vi "Copie de SaveTempData2.vi"(2 "temp data":dbl[][][](array[numeric]), 3 "Exp_params":T3={"filename"="201612011532", "ExpFilePath"=path "\\\\10.0.0.7\\takada2/DATA/HBT6/data/Test/201612011532.h5", "File Ref list"=[16777216, 33554432], "sweep_dim"=[4, 2], "sweep_list"=[], "readout_list"=["ADC0", "ADC1"], "Sweep instrument bools"=[[0, 0], [0, 0], [0, 0], [0, 0], [0, 0], [0, 0], [0, 0], [0, 0], [0, 0], [0, 0], [0, 0], [0, 0], [0, 0], [0, 0], [0, 0], [0, 0], [0, 0], [0, 0], [0, 0], [0, 0], [0, 0], [0, 0], [0, 0], [0, 0], [0, 0], [0, 0], [0, 0], [0, 0], [0, 0], [0, 0], [0, 0]], "Read out instrument bools"=[[1, 0]], "Experimental bool list"=[FALSE, TRUE], "Initial move"=[{"Name"="None", "kind"=100, "Value"=0.0}], "FPGA Ref"=refnum, "Inst_parameters"={"ConfigFilePath"=path "\\\\10.0.0.7\\takada2/DATA/HBT6/data/Configs/HBT6_ramp_1.h5", "Inst_list"=["ADC", "AWG", "Freq", "Power", "sus", "rus", "rls", "sls", "suq", "suu", "sur", "suc", "sul", "ruq", "ruu", "rur", "ruc", "rul", "rlq", "rlu", "rlr", "rlc", "rll", "slq", "slu", "slr", "slc", "sll", "tu", "t", "tl", "fast_sequence"], "fast_mode"=[1, 1], "Wait_times"=[1, 1, 1, 1], "Inst_array"=[{"Kind"=0, "Strings"=["ADC", "", "V", "ADC0;ADC1", "V;V", "1.0;1.0"], "uint64s"=[10, 2, 250000, 0, 100, 10106, 1000000, 1, 0, 1], "Doubles"=[1.0], "DAQmx take out list"=[]}, {"Kind"=7, "Strings"=["AWG", "10.0.0.4", "", "C:\\Documents and Settings\\Bauerle\\Mes documents\\Bautze\\FPGA-clean_works_1.13.6_batchtest\\Python\\AWG", "dummy", "SAWnstrig_v4.py"], "uint64s"=[2, 0, 0, 3, 0, 0, 0, 0, 0, 0, 0, 0, 0, 0], "Doubles"=[1200000000.0, 1.0, 0.0, 1.0, 0.0, 1.0, 0.0, 1.0, 0.0, 1.0, 0.0, 1.0, 0.0], "DAQmx take out list"=[]}, {"Kind"=6, "Strings"=["Freq", "0:19", "GHz"], "uint64s"=[1, 0, 0, 0, 2, 0, 0, 0], "Doubles"=[2.0, -30.0, 200.0, 100.0, 0.0, 6.000999927520752, 9.000000318337698e-06, 30.0, -145.0], "DAQmx take out list"=[]}, {"Kind"=6, "Strings"=["Power", "0:19", "GHz"], "uint64s"=[1, 0, 1, 0, 2, 0, 0, 0], "Doubles"=[2.0, -30.0, 200.0, 100.0, 0.0, 6.000999927520752, 9.000000318337698e-06, 30.0, -145.0], "DAQmx take out list"=[]}, {"Kind"=4, "Strings"=["sus", "10.0.0.2", "mV"], "uint64s"=[0, 1], "Doubles"=[1.0, -1.0, 1.0, -1.0, 1.0], "DAQmx take out list"=[]}, {"Kind"=4, "Strings"=["rus", "10.0.0.2", "mV"], "uint64s"=[0, 2], "Doubles"=[1.0, -1.0, 1.0, -1.0, 1.0], "DAQmx take out list"=[]}, {"Kind"=4, "Strings"=["rls", "10.0.0.2", "mV"], "uint64s"=[0, 3], "Doubles"=[1.0, -1.0, 1.0, -1.0, 1.0], "DAQmx take out list"=[]}, {"Kind"=4, "Strings"=["sls", "10.0.0.2", "mV"], "uint64s"=[0, 4], "Doubles"=[1.0, -1.0, 1.0, -1.0, 1.0], "DAQmx take out list"=[]}, {"Kind"=4, "Strings"=["suq", "10.0.0.2", "V"], "uint64s"=[0, 5], "Doubles"=[0.30000001192092896, -2.0, 1.0, -1.0, 1.0], "DAQmx take out list"=[]}, {"Kind"=4, "Strings"=["suu", "10.0.0.2", "V"], "uint64s"=[0, 6], "Doubles"=[0.30000001192092896, -2.0, 1.0, -1.0, 1.0], "DAQmx take out list"=[]}, {"Kind"=4, "Strings"=["sur", "10.0.0.2", "V"], "uint64s"=[0, 7], "Doubles"=[0.30000001192092896, -2.0, 1.0, -1.0, 1.0], "DAQmx take out list"=[]}, {"Kind"=4, "Strings"=["suc", "10.0.0.2", "V"], "uint64s"=[1, 0], "Doubles"=[0.30000001192092896, -2.0, 1.0, -1.0, 1.0], "DAQmx take out list"=[]}, {"Kind"=4, "Strings"=["sul", "10.0.0.2", "V"], "uint64s"=[1, 1], "Doubles"=[0.30000001192092896, -2.0, 1.0, -1.0, 1.0], "DAQmx take out list"=[]}, {"Kind"=4, "Strings"=["ruq", "10.0.0.2", "V"], "uint64s"=[1, 2], "Doubles"=[0.30000001192092896, -2.0, 1.0, -1.0, 1.0], "DAQmx take out list"=[]}, {"Kind"=4, "Strings"=["ruu", "10.0.0.2", "V"], "uint64s"=[1, 3], "Doubles"=[0.30000001192092896, -2.0, 1.0, -1.0, 1.0], "DAQmx take out list"=[]}, {"Kind"=4, "Strings"=["rur", "10.0.0.2", "V"], "uint64s"=[1, 5], "Doubles"=[0.30000001192092896, -2.0, 1.0, -1.0, 1.0], "DAQmx take out list"=[]}, {"Kind"=4, "Strings"=["ruc", "10.0.0.2", "V"], "uint64s"=[1, 6], "Doubles"=[0.30000001192092896, -2.0, 1.0, -1.0, 1.0], "DAQmx take out list"=[]}, {"Kind"=4, "Strings"=["rul", "10.0.0.2", "V"], "uint64s"=[1, 7], "Doubles"=[0.30000001192092896, -2.0, 1.0, -1.0, 1.0], "DAQmx take out list"=[]}, {"Kind"=4, "Strings"=["rlq", "10.0.0.2", "V"], "uint64s"=[2, 0], "Doubles"=[0.30000001192092896, -2.0, 1.0, -1.0, 1.0], "DAQmx take out list"=[]}, {"Kind"=4, "Strings"=["rlu", "10.0.0.2", "V"], "uint64s"=[2, 1], "Doubles"=[0.30000001192092896, -2.0, 1.0, -1.0, 1.0], "DAQmx take out list"=[]}, {"Kind"=4, "Strings"=["rlr", "10.0.0.2", "V"], "uint64s"=[2, 2], "Doubles"=[0.30000001192092896, -2.0, 1.0, -1.0, 1.0], "DAQmx take out list"=[]}, {"Kind"=4, "Strings"=["rlc", "10.0.0.2", "V"], "uint64s"=[2, 3], "Doubles"=[0.30000001192092896, -2.0, 1.0, -1.0, 1.0], "DAQmx take out list"=[]}, {"Kind"=4, "Strings"=["rll", "10.0.0.2", "V"], "uint64s"=[2, 4], "Doubles"=[0.30000001192092896, -2.0, 1.0, -1.0, 1.0], "DAQmx take out list"=[]}, {"Kind"=4, "Strings"=["slq", "10.0.0.2", "V"], "uint64s"=[2, 5], "Doubles"=[0.30000001192092896, -2.0, 1.0, -1.0, 1.0], "DAQmx take out list"=[]}, {"Kind"=4, "Strings"=["slu", "10.0.0.2", "V"], "uint64s"=[2, 6], "Doubles"=[0.30000001192092896, -2.0, 1.0, -1.0, 1.0], "DAQmx take out list"=[]}, {"Kind"=4, "Strings"=["slr", "10.0.0.2", "V"], "uint64s"=[2, 7], "Doubles"=[0.30000001192092896, -2.0, 1.0, -1.0, 1.0], "DAQmx take out list"=[]}, {"Kind"=4, "Strings"=["slc", "10.0.0.2", "V"], "uint64s"=[3, 0], "Doubles"=[0.30000001192092896, -2.0, 1.0, -1.0, 1.0], "DAQmx take out list"=[]}, {"Kind"=4, "Strings"=["sll", "10.0.0.2", "V"], "uint64s"=[3, 1], "Doubles"=[0.30000001192092896, -2.0, 1.0, -1.0, 1.0], "DAQmx take out list"=[]}, {"Kind"=4, "Strings"=["tu", "10.0.0.2", "V"], "uint64s"=[3, 2], "Doubles"=[0.30000001192092896, -2.0, 1.0, -1.0, 1.0], "DAQmx take out list"=[]}, {"Kind"=4, "Strings"=["t", "10.0.0.2", "V"], "uint64s"=[3, 3], "Doubles"=[0.30000001192092896, -2.0, 1.0, -1.0, 1.0], "DAQmx take out list"=[]}, {"Kind"=4, "Strings"=["tl", "10.0.0.2", "V"], "uint64s"=[3, 4], "Doubles"=[0.30000001192092896, -2.0, 1.0, -1.0, 1.0], "DAQmx take out list"=[]}, {"Kind"=9, "Strings"=["fast_sequence", "10.0.0.2", "V"], "uint64s"=[6661, 300, 200, 0, 0, 1, 2, 3, 4, 5, 6, 7, 16, 17, 18, 19, 20, 21, 22, 23, 0], "Doubles"=[0.5, -0.5, -1.0, -1.0], "DAQmx take out list"=[]}]}} {"File Ref list" format="%.0x"}, 4 "count":i32) -> (0 "count out":i32, 1 "Exp_params out":T3 {"File Ref list" format="%.0x"})   [LabVIEW 2010]
uses:
  <vilib>/addons/h5labview2/base/hid_t.ctl
  fpga-bitfile-ref.ctl
  <vilib>/addons/h5labview2/dataset/H5Dwrite.llb/H5Dwrite.xnode
  <vilib>/addons/h5labview2/base/lib_path.vi
  <vilib>/addons/h5labview2/base/H5Equery.vi
  <vilib>/addons/h5labview2/dataset/H5D.lvlib
  <vilib>/addons/h5labview2/space/H5S.lvlib
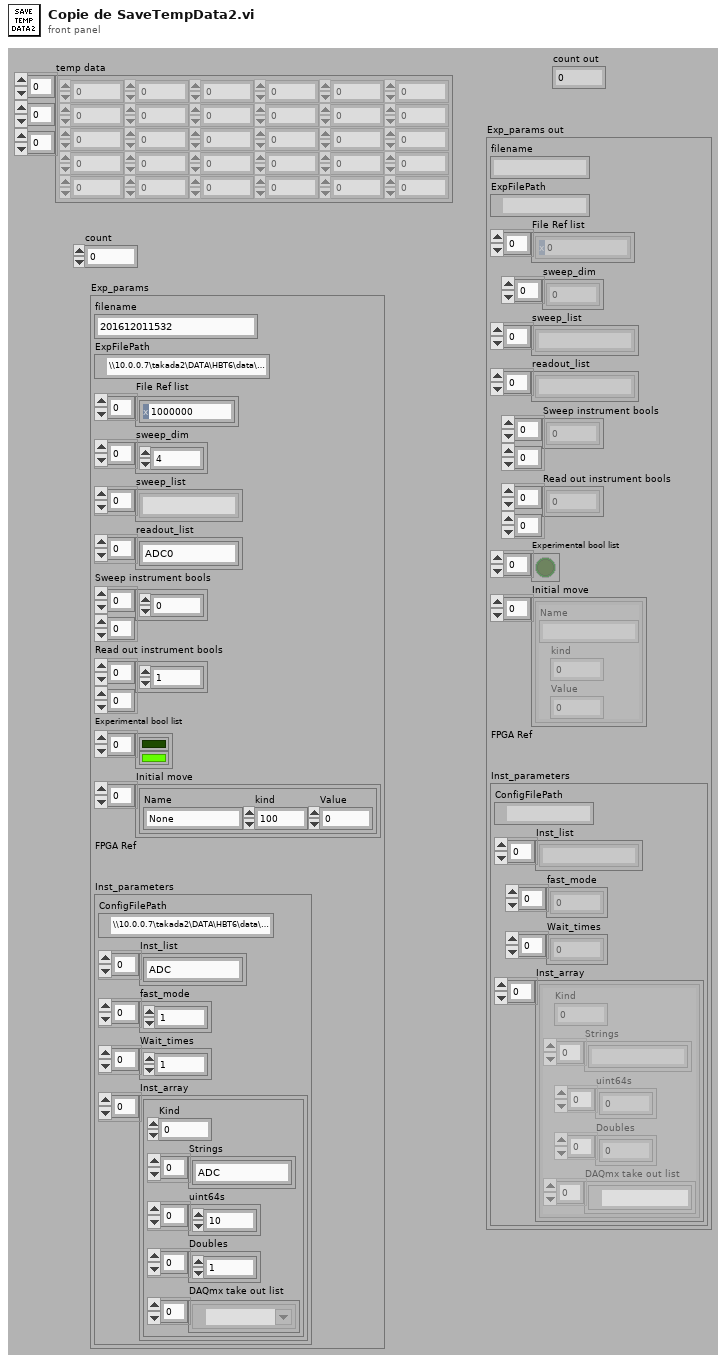
[diagram p1: front panel]
types:
  T1 = typedef "hid_t.ctl" = i32
  T2 = typedef "fpga-bitfile-ref.ctl" = refnum<k20>
  T3 = cluster{"filename":string, "ExpFilePath":path, "File Ref list":T1[], "sweep_dim":u64[], "sweep_list":string[], "readout_list":string[], "Sweep instrument bools":u64[][], "Read out instrument bools":u64[][], "Experimental bool list":bool[], "Initial move":cluster{"Name":string, "kind":u64, "Value":dbl}[], "FPGA Ref":T2, "Inst_parameters":cluster{"ConfigFilePath":path, "Inst_list":string[], "fast_mode":u8[], "Wait_times":u64[], "Inst_array":cluster{"Kind":u16, "Strings":string[], "uint64s":u64[], "Doubles":dbl[], "DAQmx take out list":refnum<k21>[]}[]}}
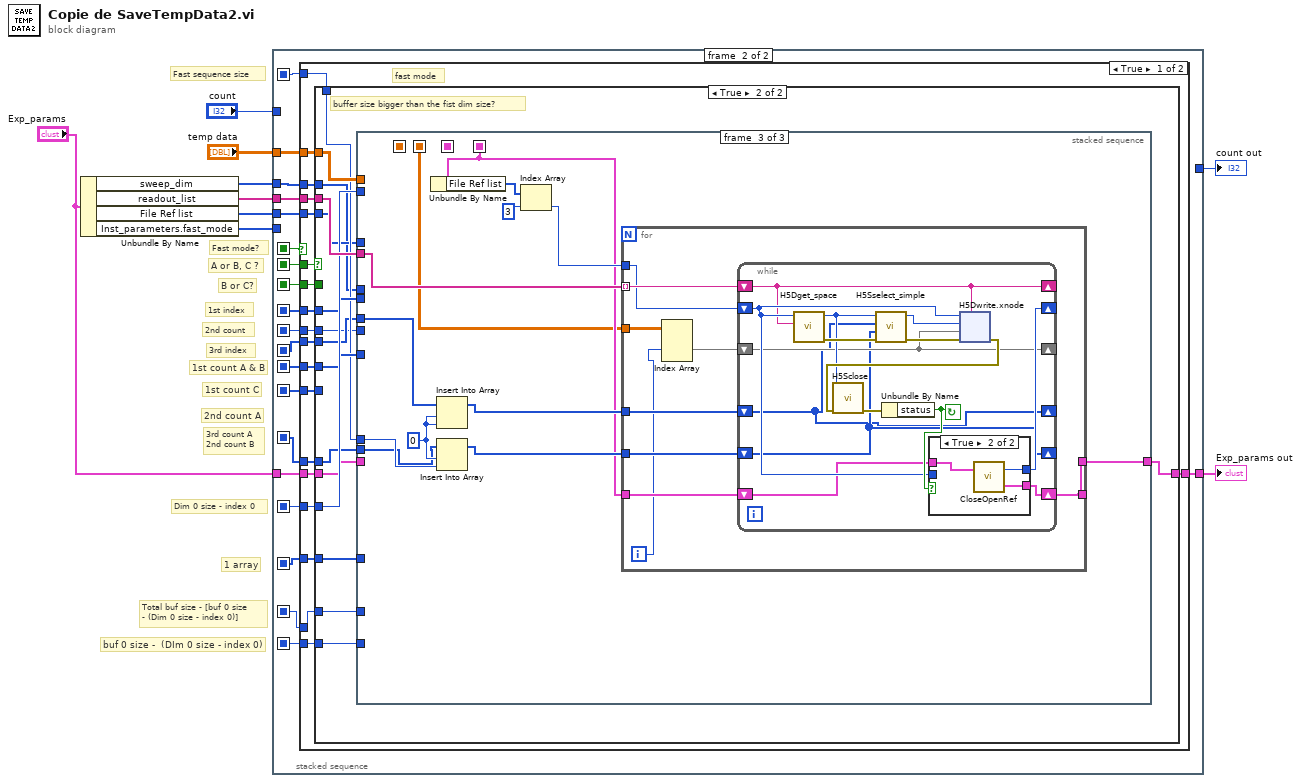
[diagram p0: block diagram]
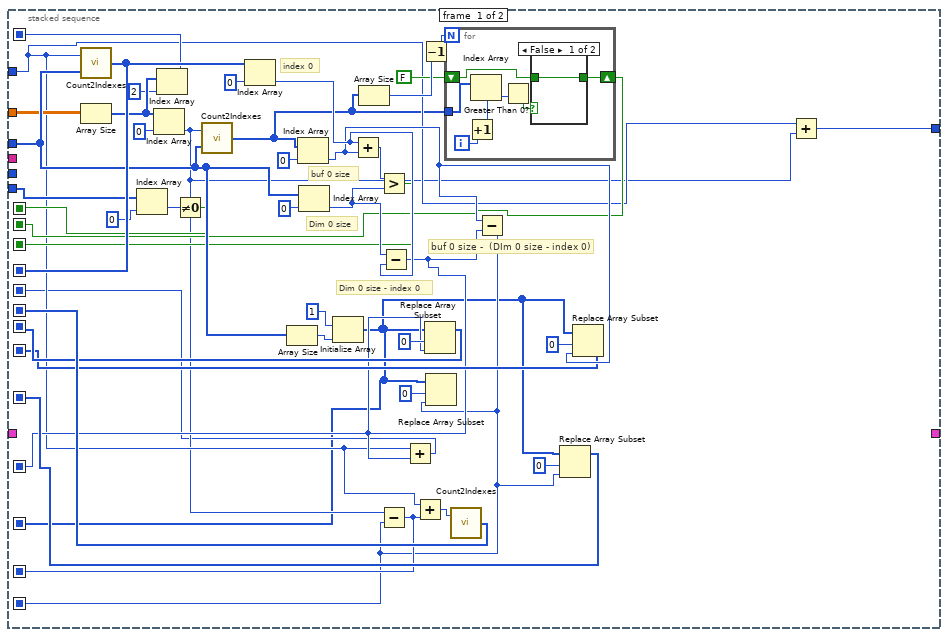
[diagram p2: hidden frame]
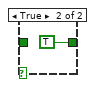
[diagram p3: hidden frame]
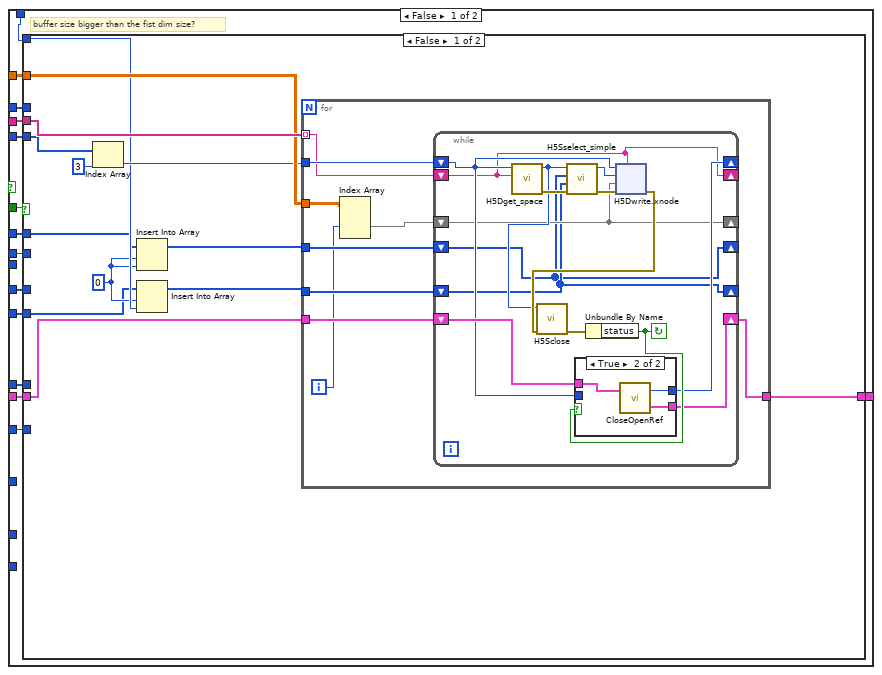
[diagram p4: hidden frame]
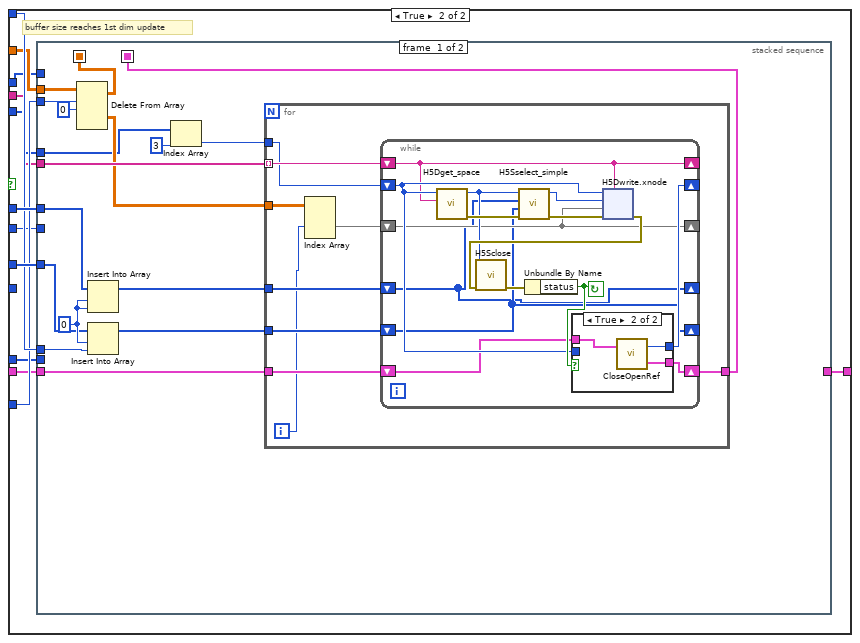
[diagram p6: hidden frame]
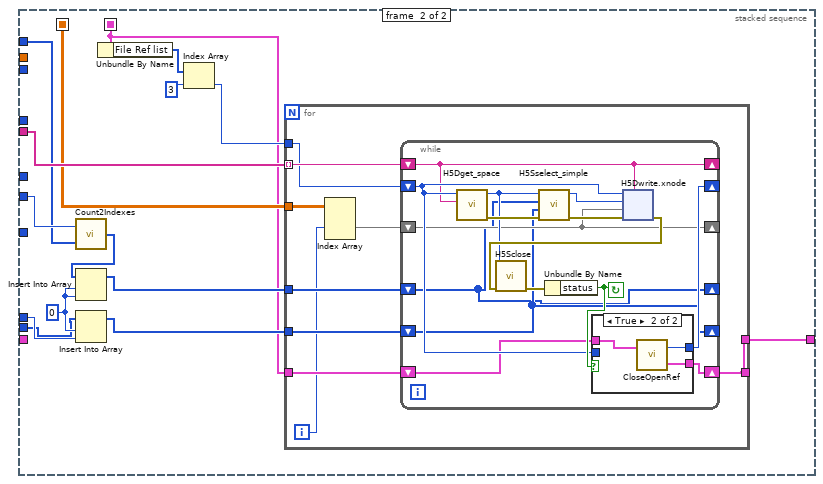
[diagram p8: hidden frame]
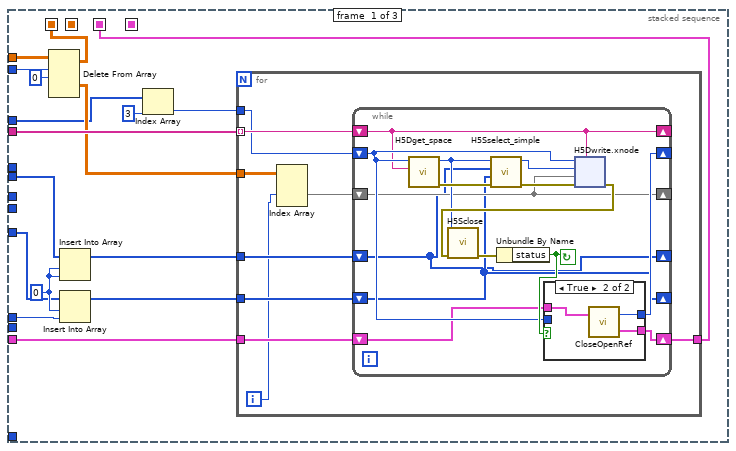
[diagram p10: hidden frame]
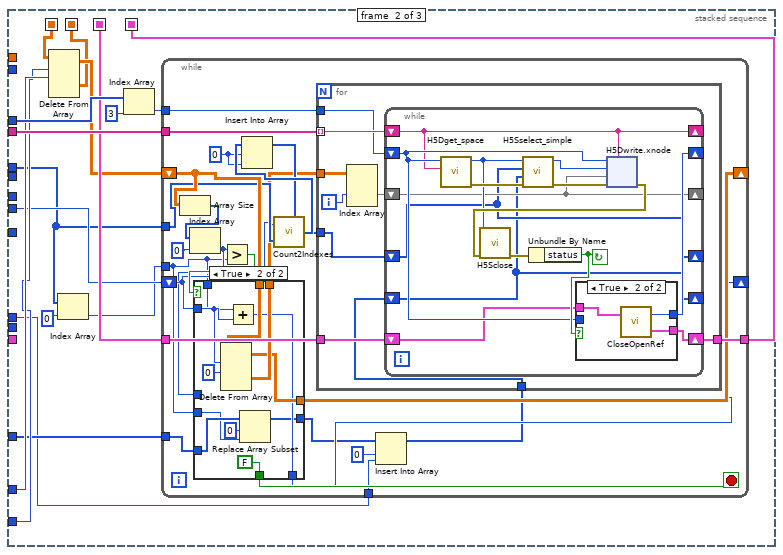
[diagram p12: hidden frame]
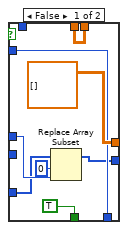
[diagram p13: hidden frame]
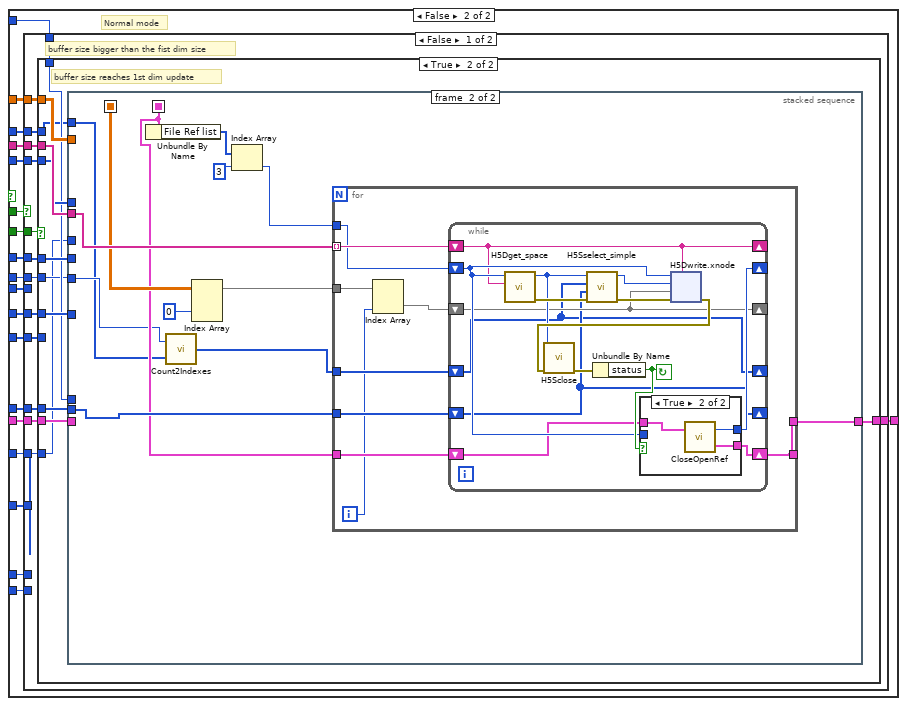
[diagram p16: hidden frame]
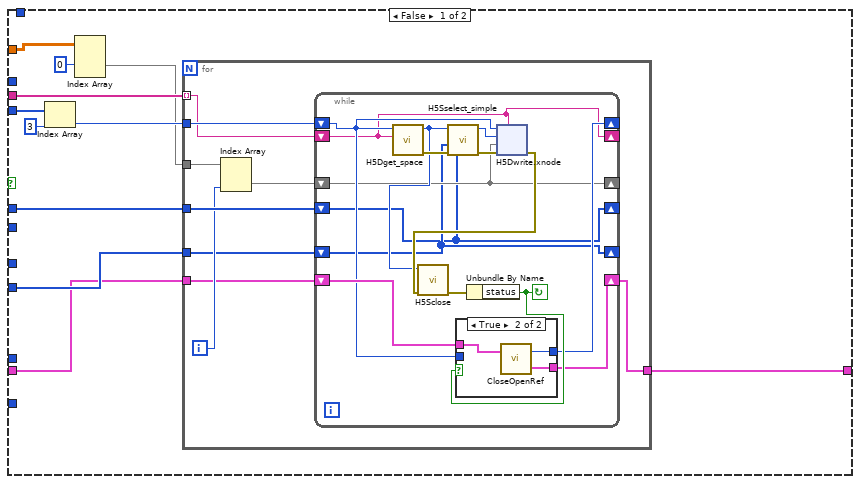
[diagram p17: hidden frame]
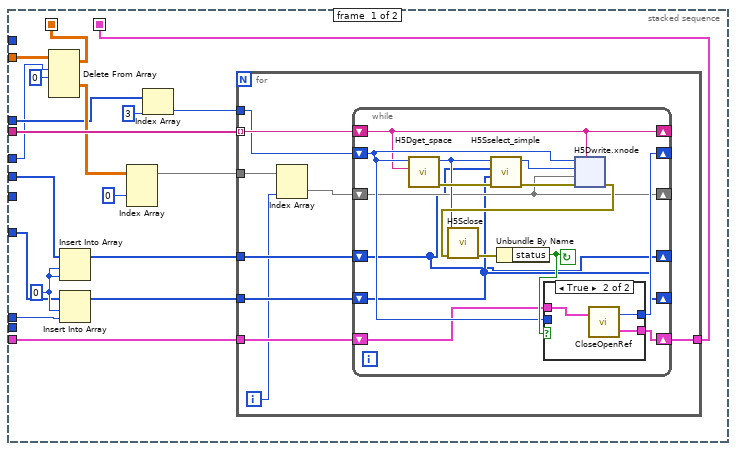
[diagram p19: hidden frame]
diagram:
  # "1 array"
  # "buf 0 size -  (DIm 0 size - index 0)"
  # "Total buf size - [buf 0 size\n- (Dim 0 size - index 0)]"
  # "Dim 0 size - index 0"
  # "Fast sequence size"
  # "B or C?"
  # "A or B, C ?"
  # "Fast mode?"
  # "3rd count A\n2nd count B"
  # "2nd count A"
  # "1st count C"
  # "1st count A & B"
  # "3rd index"
  # "2nd count"
  # "1st index"
  n1 = Unbundle By Name("Exp_params") -> ("sweep_dim"=w6:u64[], "readout_list"=w5:string[], "File Ref list"=w7:T1[], "Inst_parameters.fast_mode"=w4:u8[])
  n2 = stacked-sequence {
    seq-local: [w48 _] -> [_ w75]
    seq-local: [w11 _] -> [_ w67]
    seq-local: [w36 _] -> [_ w66]
    seq-local: [w35 _] -> [_ w71]
    seq-local: [w32 _] -> [_ w74]
    seq-local: [w29 _] -> [_ w68]
    seq-local: [w22 _] -> [_ w81]
    seq-local: [w26 _] -> [_ w80]
    seq-local: [w27 _] -> [_ w79]
    seq-local: [w19 _] -> [_ w72]
    seq-local: [w18 _] -> [_ w70]
    seq-local: [w14 _] -> [_ w65]
    seq-local: [w13 _] -> [_ w64]
    seq-local: [w10 _] -> [_ w62]
    tunnel: "count" -> [w17 _]
    tunnel: "temp data" -> [w28 w78]
    tunnel: w7 -> [_ w76]
    tunnel: w6 -> [w38 w63]
    tunnel: w5 -> [_ w77]
    tunnel: w4 -> [w25 _]
    tunnel: "Exp_params" -> [_ w73]
    tunnel: [_ w69] -> w1
    tunnel: [w16 _] -> w2
    frame #0 {
      # "buf 0 size -  (DIm 0 size - index 0)"
      # "Dim 0 size - index 0"
      # "Dim 0 size"
      # "buf 0 size"
      # "index 0"
      n3 = call "Count2Indexes.vi"("sweep_dim"=w38, "Count"=w17) -> ("Indexes"=w48:u64[])
      n4 = Array Size(array=w28) -> (size(s)=w21:i32[])
      n5 = Index Array(array=w25, index=0) -> (element=w23:u8)
      n6 = Index Array(array=w21, index=0) -> (element=w15:i32)
      n7 = Index Array(array=w21, index=2) -> (element=w19:i32)
      n8 = Not Equal To 0?(x=w23) -> (x != 0?=w22:bool)
      n9 = call "Count2Indexes.vi"("sweep_dim"=w38, "Count"=w15) -> ("Indexes"=w12:u64[])
      n10 = Index Array(array=w48, index=0) -> (element=w43:u64)
      n11 = Array Size(array=w38) -> (size(s)=w42:i32)
      n12 = Index Array(array=w12, index=0) -> (element=w33:u64)
      n13 = Index Array(array=w38, index=0) -> (element=w31:u64)
      n14 = Initialize Array(1, w42) -> (w10:i32[])
      n15 = Add(x=w43, y=w33) -> (x+y=w47:u64)
      n16 = Array Size(array=w12) -> (size(s)=w46:i32)
      n17 = Greater?(x=w47, y=w31) -> (0:w27:bool)
      n18 = Subtract(x=w31, y=w43) -> (x-y=w18:u64)
      n19 = Add(x=w17, y=w18) -> (x+y=w11:u64)
      n20 = Decrement(x=w46) -> (x-1=w45:i32)
      n21 = Replace Array Subset(array=w10, new element=w18, index=0) -> (w35:i32[])
      n22 = for {
        N: w45 -> [_]
        tunnel: w12 -> [w59]
        shift-right: [w53] -> w26
        shift-left: FALSE -> [w54]
        i -> [w58]
        n23 = Increment(x=w58) -> (x+1=w57:i32)
        n24 = Index Array(array=w59, index=w57) -> (element=w56:u64)
        n25 = Greater Than 0?(x=w56) -> (x > 0?=w55:bool)
        n26 = case shown="False" w55 {
          tunnel: w54 -> [w60 _]
          tunnel: [w60 TRUE] -> w53
          frame False {
          }
          frame True {
          }
        }
      }
      n27 = Subtract(x=w33, y=w18) -> (x-y=w13:u64)
      n28 = Subtract(x=w15, y=w13) -> (x-y=w14:u64)
      n29 = Add(x=w17, y=w14) -> (x+y=w37:u64)
      n30 = Replace Array Subset(array=w10, new element=w13, index=0) -> ()  [unwired: 1 out]
      n31 = call "Count2Indexes.vi"("Count"=w37) -> ("Indexes"=w36:u64[])  [unwired: 1 in]
      n32 = Replace Array Subset(array=w10, new element=w13, index=0) -> (w29:i32[])
      n33 = Replace Array Subset(array=w10, new element=w33, index=0) -> (w32:i32[])
      n34 = Add(x=w17, y=w15) -> (x+y=w16:i32)
    }
    frame #1 {
      n35 = case shown="True" w81 {
        tunnel: w80 -> [w100 w579]
        tunnel: w79 -> [w99 w578]
        tunnel: w78 -> [w97 w577]
        tunnel: w77 -> [w98 w576]
        tunnel: w76 -> [w96 w575]
        tunnel: w75 -> [w93 w574]
        tunnel: w74 -> [w92 w573]
        tunnel: w73 -> [w95 w572]
        tunnel: w72 -> [w94 w569]
        tunnel: w71 -> [w91 w570]
        tunnel: w70 -> [w90 w566]
        tunnel: [w89 w571] -> w69
        tunnel: w68 -> [w88 w568]
        tunnel: w67 -> [w87 w567]
        tunnel: w66 -> [w86 w561]
        tunnel: w65 -> [w85 w565]
        tunnel: w64 -> [w84 w564]
        tunnel: w63 -> [w83 w563]
        tunnel: w62 -> [w82 w562]
        frame True {
          # "fast mode"
          n36 = case shown="True" w100 {
            tunnel: w99 -> [w114 _]
            tunnel: w98 -> [w113 w327]
            tunnel: w97 -> [w112 w328]
            tunnel: w96 -> [w111 w319]
            tunnel: w95 -> [w110 w322]
            tunnel: w94 -> [w109 w323]
            tunnel: w93 -> [w108 w325]
            tunnel: w92 -> [w107 _]
            tunnel: w91 -> [w106 w324]
            tunnel: w90 -> [w105 w326]
            tunnel: [w104 w317] -> w89
            tunnel: w88 -> [w103 w320]
            tunnel: w87 -> [w102 w318]
            tunnel: w86 -> [_ w321]
            tunnel: w85 -> [_ w316]
            tunnel: w84 -> [_ w315]
            tunnel: w83 -> [w101 w314]
            tunnel: w82 -> [_ w313]
            frame False {
              # "buffer size bigger than the fist dim size?"
              n37 = case shown="False" w114 {
                tunnel: w113 -> [w127 w181]
                tunnel: w112 -> [w126 w183]
                tunnel: w111 -> [w124 w180]
                tunnel: w110 -> [w122 w179]
                tunnel: w109 -> [w121 w184]
                tunnel: w108 -> [w119 w185]
                tunnel: w107 -> [w118 _]
                tunnel: w106 -> [_ w186]
                tunnel: w105 -> [_ w182]
                tunnel: [w115 w176] -> w104
                tunnel: w103 -> [_ w178]
                tunnel: w102 -> [_ w177]
                tunnel: w101 -> [_ w175]
                frame False {
                  w120 = 0
                  n38 = Index Array(array=w124, index=3) -> (element=w123:T1)
                  n39 = Insert Into Array(array=w119, index=w120, new element=w120) -> (w117:u64[])
                  n40 = Insert Into Array(array=w118, index=w120, new element=w121) -> (w116:i32[])
                  n41 = for {
                    tunnel: w117 -> [w136]
                    tunnel: w123 -> [w135]
                    tunnel: w127 -> [w134] mode=indexing
                    tunnel: w126 -> [w133]
                    tunnel: w116 -> [w131]
                    tunnel: w122 -> [w130]
                    tunnel: [w129] -> w115
                    i -> [w128]
                    n42 = Index Array(array=w133, index (dim 1)=w128) -> (element=w132:dbl[][])  [unwired: 2 in]
                    n43 = while {
                      shift-right: [w137] -> _
                      shift-left: w136 -> [w137]
                      shift-right: [w142] -> _
                      shift-left: w135 -> [w143]
                      shift-right: [w141] -> _
                      shift-left: w132 -> [w141]
                      shift-right: [w138] -> _
                      shift-left: w131 -> [w138]
                      shift-right: [w139] -> w129
                      shift-left: w130 -> [w144]
                      shift-right: [w140] -> _
                      shift-left: w134 -> [w140]
                      stop <- w145 continue-if-true
                      n44 = call <vilib>:"H5Dget_space.vi"("obj (.)"=w140, "ref in"=w143) -> ("error out"=w151:errorcluster, "space out"=w146:T1)  [unwired: 8 in]
                      n45 = call <vilib>:"H5Sselect_simple.vi"("error in (no error)"=w151, "count"=w138, "start"=w137, "space in"=w146) -> ("error out"=w150:errorcluster, "space out"=w149:T1)  [unwired: 6 in]
                      n46 = xnode "H5Dwrite.xnode"("dataset name"=w140, "error in (no error)"=w150, "data"=w141, "file space"=w149, "ref in"=w143) -> ("error out"=w147:errorcluster)  [unwired: 2 in, 2 out]
                      n47 = call <vilib>:"H5Sclose.vi"("error in (no error)"=w147, "space in"=w146) -> ("error out"=w148:errorcluster)  [unwired: 9 in]
                      n48 = Unbundle By Name(w148) -> ("status"=w145:bool)
                      n49 = case shown="True" w145 {
                        tunnel: w143 -> [w153 _]
                        tunnel: [w153 w155] -> w142
                        tunnel: w144 -> [w152 w156]
                        tunnel: [w152 w154] -> w139
                        frame False {
                        }
                        frame True {
                          n50 = call "CloseOpenRef.vi"("Exp_params"=w156) -> ("Exp_params_out"=w154:T3, "group out"=w155:T1)  [unwired: 1 in]
                        }
                      }
                    }
                  }
                }
                frame True {
                  # "buffer size reaches 1st dim update"
                  n51 = stacked-sequence {
                    seq-local: [w196 _] -> [_ w261]
                    seq-local: [w187 _] -> [_ w254]
                    tunnel: w186 -> [w202 _]
                    tunnel: w185 -> [w201 _]
                    tunnel: w184 -> [w200 w259]
                    tunnel: w183 -> [w199 _]
                    tunnel: w182 -> [w198 _]
                    tunnel: w181 -> [w195 w265]
                    tunnel: w180 -> [w192 _]
                    tunnel: w179 -> [w188 _]
                    tunnel: w178 -> [_ w256]
                    tunnel: w177 -> [_ w253]
                    tunnel: [_ w255] -> w176
                    tunnel: w175 -> [_ w251]
                    frame #0 {
                      w203 = 0
                      n52 = Delete From Array(array=w199, length=w198, index (dim 0)=0) -> (deleted portion=w194:dbl[][][], array with subset deleted=w196:dbl[][][])  [unwired: 2 in]
                      n53 = Insert Into Array(array=w201, index=w203, new element=w203) -> (w189:u64[])
                      n54 = Insert Into Array(array=w202, index=w203, new element=w200) -> (w190:i32[])
                      n55 = Index Array(array=w192, index=3) -> (element=w191:T1)
                      n56 = for {
                        tunnel: w195 -> [w210] mode=indexing
                        tunnel: w194 -> [w212]
                        tunnel: w191 -> [w209]
                        tunnel: w190 -> [w208]
                        tunnel: w189 -> [w207]
                        tunnel: w188 -> [w206]
                        tunnel: [w205] -> w187
                        i -> [w204]
                        n57 = Index Array(array=w212, index (dim 1)=w204) -> (element=w211:dbl[][])  [unwired: 2 in]
                        n58 = while {
                          shift-right: [w218] -> _
                          shift-left: w211 -> [w218]
                          shift-right: [w213] -> _
                          shift-left: w210 -> [w213]
                          shift-right: [w219] -> _
                          shift-left: w209 -> [w220]
                          shift-right: [w216] -> w205
                          shift-left: w206 -> [w217]
                          shift-right: [w215] -> _
                          shift-left: w208 -> [w215]
                          shift-right: [w214] -> _
                          shift-left: w207 -> [w214]
                          stop <- w221 continue-if-true
                          n59 = call <vilib>:"H5Dget_space.vi"("obj (.)"=w213, "ref in"=w220) -> ("error out"=w227:errorcluster, "space out"=w222:T1)  [unwired: 8 in]
                          n60 = call <vilib>:"H5Sselect_simple.vi"("error in (no error)"=w227, "count"=w215, "start"=w214, "space in"=w222) -> ("error out"=w226:errorcluster, "space out"=w225:T1)  [unwired: 6 in]
                          n61 = xnode "H5Dwrite.xnode"("dataset name"=w213, "error in (no error)"=w226, "data"=w218, "file space"=w225, "ref in"=w220) -> ("error out"=w223:errorcluster)  [unwired: 2 in, 2 out]
                          n62 = call <vilib>:"H5Sclose.vi"("error in (no error)"=w223, "space in"=w222) -> ("error out"=w224:errorcluster)  [unwired: 9 in]
                          n63 = Unbundle By Name(w224) -> ("status"=w221:bool)
                          n64 = case shown="True" w221 {
                            tunnel: w220 -> [w229 _]
                            tunnel: [w229 w231] -> w219
                            tunnel: w217 -> [w228 w232]
                            tunnel: [w228 w230] -> w216
                            frame False {
                            }
                            frame True {
                              n65 = call "CloseOpenRef.vi"("Exp_params"=w232) -> ("Exp_params_out"=w230:T3, "group out"=w231:T1)  [unwired: 1 in]
                            }
                          }
                        }
                      }
                    }
                    frame #1 {
                      w260 = 0
                      n66 = call "Count2Indexes.vi"("sweep_dim"=w251, "Count"=w253) -> ("Indexes"=w252:u64[])
                      n67 = Insert Into Array(array=w252, index=w260, new element=w260) -> (w257:u64[])
                      n68 = Insert Into Array(array=w256, index=w260, new element=w259) -> (w258:i32[])
                      n69 = Unbundle By Name(w254) -> ("File Ref list"=w264:T1[])
                      n70 = Index Array(array=w264, index=3) -> (element=w262:T1)
                      n71 = for {
                        tunnel: w265 -> [w272] mode=indexing
                        tunnel: w261 -> [w274]
                        tunnel: w262 -> [w271]
                        tunnel: w258 -> [w270]
                        tunnel: w257 -> [w269]
                        tunnel: w254 -> [w268]
                        tunnel: [w267] -> _
                        tunnel: [w267] -> w255
                        i -> [w266]
                        n72 = Index Array(array=w274, index (dim 1)=w266) -> (element=w273:dbl[][])  [unwired: 2 in]
                        n73 = while {
                          shift-right: [w280] -> _
                          shift-left: w273 -> [w280]
                          shift-right: [w275] -> _
                          shift-left: w272 -> [w275]
                          shift-right: [w281] -> _
                          shift-left: w271 -> [w282]
                          shift-right: [w278] -> w267
                          shift-left: w268 -> [w279]
                          shift-right: [w277] -> _
                          shift-left: w270 -> [w277]
                          shift-right: [w276] -> _
                          shift-left: w269 -> [w276]
                          stop <- w283 continue-if-true
                          n74 = call <vilib>:"H5Dget_space.vi"("obj (.)"=w275, "ref in"=w282) -> ("error out"=w289:errorcluster, "space out"=w284:T1)  [unwired: 8 in]
                          n75 = call <vilib>:"H5Sselect_simple.vi"("error in (no error)"=w289, "count"=w277, "start"=w276, "space in"=w284) -> ("error out"=w288:errorcluster, "space out"=w287:T1)  [unwired: 6 in]
                          n76 = xnode "H5Dwrite.xnode"("dataset name"=w275, "error in (no error)"=w288, "data"=w280, "file space"=w287, "ref in"=w282) -> ("error out"=w285:errorcluster)  [unwired: 2 in, 2 out]
                          n77 = call <vilib>:"H5Sclose.vi"("error in (no error)"=w285, "space in"=w284) -> ("error out"=w286:errorcluster)  [unwired: 9 in]
                          n78 = Unbundle By Name(w286) -> ("status"=w283:bool)
                          n79 = case shown="True" w283 {
                            tunnel: w282 -> [w291 _]
                            tunnel: [w291 w293] -> w281
                            tunnel: w279 -> [w290 w294]
                            tunnel: [w290 w292] -> w278
                            frame False {
                            }
                            frame True {
                              n80 = call "CloseOpenRef.vi"("Exp_params"=w294) -> ("Exp_params_out"=w292:T3, "group out"=w293:T1)  [unwired: 1 in]
                            }
                          }
                        }
                      }
                    }
                  }
                }
              }
            }
            frame True {
              # "buffer size bigger than the fist dim size?"
              n81 = stacked-sequence {
                seq-local: [w338 _ _] -> [_ w403 _]
                seq-local: [w329 _ _] -> [_ w405 _]
                seq-local: [_ w404 _] -> [_ _ w502]
                seq-local: [_ w401 _] -> [_ _ w501]
                tunnel: w324 -> [w344 _ _]
                tunnel: w325 -> [w343 _ _]
                tunnel: w323 -> [w342 w393 w508]
                tunnel: w328 -> [w341 _ _]
                tunnel: w326 -> [w340 _ _]
                tunnel: w327 -> [w337 w409 w513]
                tunnel: w319 -> [w334 w407 _]
                tunnel: w322 -> [w330 _ _]
                tunnel: w320 -> [_ _ w505]
                tunnel: w321 -> [_ _ w504]
                tunnel: [_ _ w503] -> w317
                tunnel: w318 -> [_ w398 _]
                tunnel: w316 -> [_ w400 _]
                tunnel: w315 -> [_ w399 _]
                tunnel: w314 -> [_ w397 _]
                tunnel: w313 -> [_ w394 _]
                frame #0 {
                  w345 = 0
                  n82 = Delete From Array(array=w341, length=w340, index (dim 0)=0) -> (deleted portion=w336:dbl[][][], array with subset deleted=w338:dbl[][][])  [unwired: 2 in]
                  n83 = Insert Into Array(array=w343, index=w345, new element=w345) -> (w331:u64[])
                  n84 = Insert Into Array(array=w344, index=w345, new element=w342) -> (w332:i32[])
                  n85 = Index Array(array=w334, index=3) -> (element=w333:T1)
                  n86 = for {
                    tunnel: w337 -> [w352] mode=indexing
                    tunnel: w336 -> [w354]
                    tunnel: w333 -> [w351]
                    tunnel: w332 -> [w350]
                    tunnel: w331 -> [w349]
                    tunnel: w330 -> [w348]
                    tunnel: [w347] -> w329
                    i -> [w346]
                    n87 = Index Array(array=w354, index (dim 1)=w346) -> (element=w353:dbl[][])  [unwired: 2 in]
                    n88 = while {
                      shift-right: [w360] -> _
                      shift-left: w353 -> [w360]
                      shift-right: [w355] -> _
                      shift-left: w352 -> [w355]
                      shift-right: [w361] -> _
                      shift-left: w351 -> [w362]
                      shift-right: [w358] -> w347
                      shift-left: w348 -> [w359]
                      shift-right: [w357] -> _
                      shift-left: w350 -> [w357]
                      shift-right: [w356] -> _
                      shift-left: w349 -> [w356]
                      stop <- w363 continue-if-true
                      n89 = call <vilib>:"H5Dget_space.vi"("obj (.)"=w355, "ref in"=w362) -> ("error out"=w369:errorcluster, "space out"=w364:T1)  [unwired: 8 in]
                      n90 = call <vilib>:"H5Sselect_simple.vi"("error in (no error)"=w369, "count"=w357, "start"=w356, "space in"=w364) -> ("error out"=w368:errorcluster, "space out"=w367:T1)  [unwired: 6 in]
                      n91 = xnode "H5Dwrite.xnode"("dataset name"=w355, "error in (no error)"=w368, "data"=w360, "file space"=w367, "ref in"=w362) -> ("error out"=w365:errorcluster)  [unwired: 2 in, 2 out]
                      n92 = call <vilib>:"H5Sclose.vi"("error in (no error)"=w365, "space in"=w364) -> ("error out"=w366:errorcluster)  [unwired: 9 in]
                      n93 = Unbundle By Name(w366) -> ("status"=w363:bool)
                      n94 = case shown="True" w363 {
                        tunnel: w362 -> [w371 _]
                        tunnel: [w371 w373] -> w361
                        tunnel: w359 -> [w370 w374]
                        tunnel: [w370 w372] -> w358
                        frame False {
                        }
                        frame True {
                          n95 = call "CloseOpenRef.vi"("Exp_params"=w374) -> ("Exp_params_out"=w372:T3, "group out"=w373:T1)  [unwired: 1 in]
                        }
                      }
                    }
                  }
                }
                frame #1 {
                  n96 = Delete From Array(array=w403, length=w399, index (dim 0)=w400) -> (deleted portion=w401:dbl[][][], array with subset deleted=w402:dbl[][][])  [unwired: 2 in]
                  n97 = Index Array(array=w397, index=0) -> (element=w395:u64)
                  n98 = Index Array(array=w407, index=3) -> (element=w406:T1)
                  n99 = while {
                    tunnel: w409 -> [w433]
                    tunnel: w406 -> [w432]
                    tunnel: w405 -> [w431]
                    tunnel: [w430] -> w404
                    shift-right: [w424] -> _
                    shift-left: w402 -> [w426]
                    tunnel: w397 -> [w422]
                    shift-right: [w423] -> _
                    shift-left: w398 -> [w421]
                    tunnel: w395 -> [w415]
                    tunnel: w394 -> [w414]
                    tunnel: w393 -> [w411]
                    stop <- w425 stop-if-true
                    w419 = 0
                    n100 = Array Size(array=w426) -> (size(s)=w429:i32[])
                    n101 = Index Array(array=w429, index=0) -> (element=w416:i32)
                    n102 = Greater?(x=w416, y=w415) -> (0:w427:bool)
                    n103 = case shown="True" w427 {
                      tunnel: w421 -> [w438 w453]
                      tunnel: w415 -> [_ w449]
                      tunnel: w426 -> [w440 w452]
                      tunnel: [w440 w451] -> w417
                      tunnel: [TRUE FALSE] -> w425
                      tunnel: [dbl[][][] [] w447] -> w424
                      tunnel: [w438 w446] -> w423
                      tunnel: w416 -> [w435 _]
                      tunnel: w415 -> [_ w444]
                      tunnel: w414 -> [w434 w445]
                      tunnel: [w436 w442] -> w413
                      frame False {
                        n104 = Replace Array Subset(array=w434, new element=w435, index=0) -> (w436:i32[])
                      }
                      frame True {
                        n105 = Delete From Array(array=w452, length=w449, index (dim 0)=0) -> (deleted portion=w451:dbl[][][], array with subset deleted=w447:dbl[][][])  [unwired: 2 in]
                        n106 = Add(x=w449, y=w453) -> (x+y=w446:u64)
                        n107 = Replace Array Subset(array=w445, new element=w444, index=0) -> (w442:i32[])
                      }
                    }
                    n108 = call "Count2Indexes.vi"("sweep_dim"=w422, "Count"=w421) -> ("Indexes"=w420:u64[])
                    n109 = Insert Into Array(array=w420, index=w419, new element=w419) -> (w418:u64[])
                    n110 = Insert Into Array(array=w413, index=0, new element=w411) -> (w410:i32[])
                    n111 = for {
                      tunnel: w433 -> [w460] mode=indexing
                      tunnel: w417 -> [w462]
                      tunnel: w432 -> [w459]
                      tunnel: w431 -> [w458]
                      tunnel: [w457] -> w430
                      tunnel: w418 -> [w456]
                      tunnel: w410 -> [w455]
                      i -> [w454]
                      n112 = Index Array(array=w462, index (dim 1)=w454) -> (element=w461:dbl[][])  [unwired: 2 in]
                      n113 = while {
                        shift-right: [w468] -> _
                        shift-left: w461 -> [w468]
                        shift-right: [w465] -> _
                        shift-left: w460 -> [w465]
                        shift-right: [w469] -> _
                        shift-left: w459 -> [w470]
                        shift-right: [w466] -> w457
                        shift-left: w458 -> [w467]
                        shift-right: [w463] -> _
                        shift-left: w455 -> [w463]
                        shift-right: [w464] -> _
                        shift-left: w456 -> [w464]
                        stop <- w471 continue-if-true
                        n114 = call <vilib>:"H5Dget_space.vi"("obj (.)"=w465, "ref in"=w470) -> ("error out"=w477:errorcluster, "space out"=w472:T1)  [unwired: 8 in]
                        n115 = call <vilib>:"H5Sselect_simple.vi"("error in (no error)"=w477, "count"=w463, "start"=w464, "space in"=w472) -> ("error out"=w476:errorcluster, "space out"=w475:T1)  [unwired: 6 in]
                        n116 = xnode "H5Dwrite.xnode"("dataset name"=w465, "error in (no error)"=w476, "data"=w468, "file space"=w475, "ref in"=w470) -> ("error out"=w473:errorcluster)  [unwired: 2 in, 2 out]
                        n117 = call <vilib>:"H5Sclose.vi"("error in (no error)"=w473, "space in"=w472) -> ("error out"=w474:errorcluster)  [unwired: 9 in]
                        n118 = Unbundle By Name(w474) -> ("status"=w471:bool)
                        n119 = case shown="True" w471 {
                          tunnel: w470 -> [w479 _]
                          tunnel: [w479 w481] -> w469
                          tunnel: w467 -> [w478 w482]
                          tunnel: [w478 w480] -> w466
                          frame False {
                          }
                          frame True {
                            n120 = call "CloseOpenRef.vi"("Exp_params"=w482) -> ("Exp_params_out"=w480:T3, "group out"=w481:T1)  [unwired: 1 in]
                          }
                        }
                      }
                    }
                  }
                }
                frame #2 {
                  w509 = 0
                  n121 = Unbundle By Name(w502) -> ("File Ref list"=w512:T1[])
                  n122 = Insert Into Array(array=w504, index=w509, new element=w509) -> (w506:u64[])
                  n123 = Insert Into Array(array=w505, index=w509, new element=w508) -> (w507:i32[])
                  n124 = Index Array(array=w512, index=3) -> (element=w510:T1)
                  n125 = for {
                    tunnel: w513 -> [w520] mode=indexing
                    tunnel: w501 -> [w522]
                    tunnel: w510 -> [w519]
                    tunnel: w507 -> [w518]
                    tunnel: w506 -> [w517]
                    tunnel: w502 -> [w516]
                    tunnel: [w515] -> _
                    tunnel: [w515] -> w503
                    i -> [w514]
                    n126 = Index Array(array=w522, index (dim 1)=w514) -> (element=w521:dbl[][])  [unwired: 2 in]
                    n127 = while {
                      shift-right: [w528] -> _
                      shift-left: w521 -> [w528]
                      shift-right: [w523] -> _
                      shift-left: w520 -> [w523]
                      shift-right: [w529] -> _
                      shift-left: w519 -> [w530]
                      shift-right: [w526] -> w515
                      shift-left: w516 -> [w527]
                      shift-right: [w525] -> _
                      shift-left: w518 -> [w525]
                      shift-right: [w524] -> _
                      shift-left: w517 -> [w524]
                      stop <- w531 continue-if-true
                      n128 = call <vilib>:"H5Dget_space.vi"("obj (.)"=w523, "ref in"=w530) -> ("error out"=w537:errorcluster, "space out"=w532:T1)  [unwired: 8 in]
                      n129 = call <vilib>:"H5Sselect_simple.vi"("error in (no error)"=w537, "count"=w525, "start"=w524, "space in"=w532) -> ("error out"=w536:errorcluster, "space out"=w535:T1)  [unwired: 6 in]
                      n130 = xnode "H5Dwrite.xnode"("dataset name"=w523, "error in (no error)"=w536, "data"=w528, "file space"=w535, "ref in"=w530) -> ("error out"=w533:errorcluster)  [unwired: 2 in, 2 out]
                      n131 = call <vilib>:"H5Sclose.vi"("error in (no error)"=w533, "space in"=w532) -> ("error out"=w534:errorcluster)  [unwired: 9 in]
                      n132 = Unbundle By Name(w534) -> ("status"=w531:bool)
                      n133 = case shown="True" w531 {
                        tunnel: w530 -> [w539 _]
                        tunnel: [w539 w541] -> w529
                        tunnel: w527 -> [w538 w542]
                        tunnel: [w538 w540] -> w526
                        frame False {
                        }
                        frame True {
                          n134 = call "CloseOpenRef.vi"("Exp_params"=w542) -> ("Exp_params_out"=w540:T3, "group out"=w541:T1)  [unwired: 1 in]
                        }
                      }
                    }
                  }
                }
              }
            }
          }
        }
        frame False {
          # "Normal mode"
          n135 = case shown="False" w579 {
            tunnel: w578 -> [w593 _]
            tunnel: w577 -> [w592 w792]
            tunnel: w576 -> [w591 w803]
            tunnel: w575 -> [w590 w802]
            tunnel: w574 -> [w589 w801]
            tunnel: w573 -> [w588 _]
            tunnel: w572 -> [w587 w805]
            tunnel: [w586 w806] -> w571
            tunnel: w570 -> [w585 w800]
            tunnel: w569 -> [w584 _]
            tunnel: w568 -> [w583 w793]
            tunnel: w567 -> [w582 w796]
            tunnel: w566 -> [w581 w804]
            tunnel: w565 -> [_ w799]
            tunnel: w564 -> [_ w798]
            tunnel: w563 -> [w580 w797]
            tunnel: w562 -> [_ w795]
            tunnel: w561 -> [_ w794]
            frame False {
              # "buffer size bigger than the fist dim size"
              n136 = case shown="True" w593 {
                tunnel: w592 -> [w599 w662]
                tunnel: w591 -> [w600 w661]
                tunnel: w590 -> [w604 w660]
                tunnel: w589 -> [w602 w659]
                tunnel: w588 -> [w596 _]
                tunnel: w587 -> [w595 w656]
                tunnel: [w594 w663] -> w586
                tunnel: w585 -> [_ w658]
                tunnel: w584 -> [_ w657]
                tunnel: w583 -> [_ w655]
                tunnel: w582 -> [_ w654]
                tunnel: w581 -> [_ w653]
                tunnel: w580 -> [_ w652]
                frame False {
                  n137 = Index Array(array=w604, index=3) -> (element=w601:T1)
                  n138 = Index Array(array=w599, index (dim 1)=0) -> (element=w597:dbl[][])  [unwired: 2 in]
                  n139 = for {
                    tunnel: w602 -> [w613]
                    tunnel: w601 -> [w612]
                    tunnel: w600 -> [w611] mode=indexing
                    tunnel: w597 -> [w610]
                    tunnel: w596 -> [w607]
                    tunnel: w595 -> [w606]
                    tunnel: [w605] -> w594
                    i -> [w609]
                    n140 = Index Array(array=w610, index (col)=w609) -> (element=w608:dbl[])  [unwired: 1 in]
                    n141 = while {
                      shift-right: [w614] -> _
                      shift-left: w613 -> [w614]
                      shift-right: [w619] -> _
                      shift-left: w612 -> [w620]
                      shift-right: [w618] -> _
                      shift-left: w608 -> [w618]
                      shift-right: [w615] -> _
                      shift-left: w607 -> [w615]
                      shift-right: [w616] -> w605
                      shift-left: w606 -> [w621]
                      shift-right: [w617] -> _
                      shift-left: w611 -> [w617]
                      stop <- w622 continue-if-true
                      n142 = call <vilib>:"H5Dget_space.vi"("obj (.)"=w617, "ref in"=w620) -> ("error out"=w628:errorcluster, "space out"=w623:T1)  [unwired: 8 in]
                      n143 = call <vilib>:"H5Sselect_simple.vi"("error in (no error)"=w628, "count"=w615, "start"=w614, "space in"=w623) -> ("error out"=w627:errorcluster, "space out"=w626:T1)  [unwired: 6 in]
                      n144 = xnode "H5Dwrite.xnode"("dataset name"=w617, "error in (no error)"=w627, "data"=w618, "file space"=w626, "ref in"=w620) -> ("error out"=w624:errorcluster)  [unwired: 2 in, 2 out]
                      n145 = call <vilib>:"H5Sclose.vi"("error in (no error)"=w624, "space in"=w623) -> ("error out"=w625:errorcluster)  [unwired: 9 in]
                      n146 = Unbundle By Name(w625) -> ("status"=w622:bool)
                      n147 = case shown="True" w622 {
                        tunnel: w620 -> [w630 _]
                        tunnel: [w630 w632] -> w619
                        tunnel: w621 -> [w629 w633]
                        tunnel: [w629 w631] -> w616
                        frame False {
                        }
                        frame True {
                          n148 = call "CloseOpenRef.vi"("Exp_params"=w633) -> ("Exp_params_out"=w631:T3, "group out"=w632:T1)  [unwired: 1 in]
                        }
                      }
                    }
                  }
                }
                frame True {
                  # "buffer size reaches 1st dim update"
                  n149 = stacked-sequence {
                    seq-local: [w676 _] -> [_ w738]
                    seq-local: [w667 _] -> [_ w733]
                    tunnel: w658 -> [w681 _]
                    tunnel: w659 -> [w680 _]
                    tunnel: w657 -> [w679 _]
                    tunnel: w662 -> [w678 _]
                    tunnel: w661 -> [w675 w742]
                    tunnel: w660 -> [w672 _]
                    tunnel: w656 -> [w668 _]
                    tunnel: w655 -> [_ w736]
                    tunnel: w654 -> [_ w731]
                    tunnel: [_ w737] -> w663
                    tunnel: w653 -> [w666 _]
                    tunnel: w652 -> [_ w730]
                    frame #0 {
                      w682 = 0
                      n150 = Delete From Array(array=w678, length=w666, index (dim 0)=0) -> (deleted portion=w674:dbl[][][], array with subset deleted=w676:dbl[][][])  [unwired: 2 in]
                      n151 = Insert Into Array(array=w680, index=w682, new element=w682) -> (w669:u64[])
                      n152 = Insert Into Array(array=w681, index=w682, new element=w679) -> (w670:i32[])
                      n153 = Index Array(array=w674, index (dim 1)=0) -> (element=w665:dbl[][])  [unwired: 2 in]
                      n154 = Index Array(array=w672, index=3) -> (element=w671:T1)
                      n155 = for {
                        tunnel: w675 -> [w689] mode=indexing
                        tunnel: w665 -> [w691]
                        tunnel: w671 -> [w688]
                        tunnel: w670 -> [w687]
                        tunnel: w669 -> [w686]
                        tunnel: w668 -> [w685]
                        tunnel: [w684] -> w667
                        i -> [w683]
                        n156 = Index Array(array=w691, index (col)=w683) -> (element=w690:dbl[])  [unwired: 1 in]
                        n157 = while {
                          shift-right: [w697] -> _
                          shift-left: w690 -> [w697]
                          shift-right: [w692] -> _
                          shift-left: w689 -> [w692]
                          shift-right: [w698] -> _
                          shift-left: w688 -> [w699]
                          shift-right: [w695] -> w684
                          shift-left: w685 -> [w696]
                          shift-right: [w694] -> _
                          shift-left: w687 -> [w694]
                          shift-right: [w693] -> _
                          shift-left: w686 -> [w693]
                          stop <- w700 continue-if-true
                          n158 = call <vilib>:"H5Dget_space.vi"("obj (.)"=w692, "ref in"=w699) -> ("error out"=w706:errorcluster, "space out"=w701:T1)  [unwired: 8 in]
                          n159 = call <vilib>:"H5Sselect_simple.vi"("error in (no error)"=w706, "count"=w694, "start"=w693, "space in"=w701) -> ("error out"=w705:errorcluster, "space out"=w704:T1)  [unwired: 6 in]
                          n160 = xnode "H5Dwrite.xnode"("dataset name"=w692, "error in (no error)"=w705, "data"=w697, "file space"=w704, "ref in"=w699) -> ("error out"=w702:errorcluster)  [unwired: 2 in, 2 out]
                          n161 = call <vilib>:"H5Sclose.vi"("error in (no error)"=w702, "space in"=w701) -> ("error out"=w703:errorcluster)  [unwired: 9 in]
                          n162 = Unbundle By Name(w703) -> ("status"=w700:bool)
                          n163 = case shown="True" w700 {
                            tunnel: w699 -> [w708 _]
                            tunnel: [w708 w710] -> w698
                            tunnel: w696 -> [w707 w711]
                            tunnel: [w707 w709] -> w695
                            frame False {
                            }
                            frame True {
                              n164 = call "CloseOpenRef.vi"("Exp_params"=w711) -> ("Exp_params_out"=w709:T3, "group out"=w710:T1)  [unwired: 1 in]
                            }
                          }
                        }
                      }
                    }
                    frame #1 {
                      n165 = Unbundle By Name(w733) -> ("File Ref list"=w741:T1[])
                      n166 = call "Count2Indexes.vi"("sweep_dim"=w730, "Count"=w731) -> ("Indexes"=w732:u64[])
                      n167 = Index Array(array=w738, index (dim 1)=0) -> (element=w735:dbl[][])  [unwired: 2 in]
                      n168 = Index Array(array=w741, index=3) -> (element=w739:T1)
                      n169 = for {
                        tunnel: w742 -> [w749] mode=indexing
                        tunnel: w735 -> [w751]
                        tunnel: w739 -> [w748]
                        tunnel: w736 -> [w747]
                        tunnel: w732 -> [w746]
                        tunnel: w733 -> [w745]
                        tunnel: [w744] -> _
                        tunnel: [w744] -> w737
                        i -> [w743]
                        n170 = Index Array(array=w751, index (col)=w743) -> (element=w750:dbl[])  [unwired: 1 in]
                        n171 = while {
                          shift-right: [w757] -> _
                          shift-left: w750 -> [w757]
                          shift-right: [w753] -> _
                          shift-left: w749 -> [w753]
                          shift-right: [w758] -> _
                          shift-left: w748 -> [w759]
                          shift-right: [w755] -> w744
                          shift-left: w745 -> [w756]
                          shift-right: [w754] -> _
                          shift-left: w747 -> [w754]
                          shift-right: [w752] -> _
                          shift-left: w746 -> [w752]
                          stop <- w760 continue-if-true
                          n172 = call <vilib>:"H5Dget_space.vi"("obj (.)"=w753, "ref in"=w759) -> ("error out"=w766:errorcluster, "space out"=w761:T1)  [unwired: 8 in]
                          n173 = call <vilib>:"H5Sselect_simple.vi"("error in (no error)"=w766, "count"=w754, "start"=w752, "space in"=w761) -> ("error out"=w765:errorcluster, "space out"=w764:T1)  [unwired: 6 in]
                          n174 = xnode "H5Dwrite.xnode"("dataset name"=w753, "error in (no error)"=w765, "data"=w757, "file space"=w764, "ref in"=w759) -> ("error out"=w762:errorcluster)  [unwired: 2 in, 2 out]
                          n175 = call <vilib>:"H5Sclose.vi"("error in (no error)"=w762, "space in"=w761) -> ("error out"=w763:errorcluster)  [unwired: 9 in]
                          n176 = Unbundle By Name(w763) -> ("status"=w760:bool)
                          n177 = case shown="True" w760 {
                            tunnel: w759 -> [w768 _]
                            tunnel: [w768 w770] -> w758
                            tunnel: w756 -> [w767 w771]
                            tunnel: [w767 w769] -> w755
                            frame False {
                            }
                            frame True {
                              n178 = call "CloseOpenRef.vi"("Exp_params"=w771) -> ("Exp_params_out"=w769:T3, "group out"=w770:T1)  [unwired: 1 in]
                            }
                          }
                        }
                      }
                    }
                  }
                }
              }
            }
            frame True {
              # "buffer size smaller than the fist dim size"
              n179 = Index Array(array=w792, index (dim 1)=0) -> (element=w790:dbl[][])  [unwired: 2 in]
              n180 = stacked-sequence {
                seq-local: [w816 _ _] -> [_ w876 _]
                seq-local: [w809 _ _] -> [_ w878 _]
                seq-local: [_ w877 _] -> [_ _ w972]
                seq-local: [_ w874 _] -> [_ _ w971]
                tunnel: w800 -> [w808 _ _]
                tunnel: w801 -> [w807 _ _]
                tunnel: w790 -> [w819 _ _]
                tunnel: w804 -> [w818 _ _]
                tunnel: w803 -> [w815 w882 w977]
                tunnel: w802 -> [w812 w880 _]
                tunnel: w805 -> [w810 _ _]
                tunnel: w793 -> [_ _ w969]
                tunnel: w794 -> [_ _ w970]
                tunnel: [_ _ w973] -> w806
                tunnel: w796 -> [_ w871 _]
                tunnel: w799 -> [_ w873 _]
                tunnel: w798 -> [_ w872 _]
                tunnel: w797 -> [_ w870 _]
                tunnel: w795 -> [_ w867 _]
                frame #0 {
                  n181 = Delete From Array(array=w819, length=w818, index (row)=0) -> (deleted portion=w814:dbl[][], array with subset deleted=w816:dbl[][])  [unwired: 1 in]
                  n182 = Index Array(array=w812, index=3) -> (element=w811:T1)
                  n183 = for {
                    tunnel: w815 -> [w826] mode=indexing
                    tunnel: w814 -> [w828]
                    tunnel: w811 -> [w825]
                    tunnel: w808 -> [w824]
                    tunnel: w807 -> [w823]
                    tunnel: w810 -> [w822]
                    tunnel: [w821] -> w809
                    i -> [w820]
                    n184 = Index Array(array=w828, index (col)=w820) -> (element=w827:dbl[])  [unwired: 1 in]
                    n185 = while {
                      shift-right: [w834] -> _
                      shift-left: w827 -> [w834]
                      shift-right: [w829] -> _
                      shift-left: w826 -> [w829]
                      shift-right: [w835] -> _
                      shift-left: w825 -> [w836]
                      shift-right: [w832] -> w821
                      shift-left: w822 -> [w833]
                      shift-right: [w831] -> _
                      shift-left: w824 -> [w831]
                      shift-right: [w830] -> _
                      shift-left: w823 -> [w830]
                      stop <- w837 continue-if-true
                      n186 = call <vilib>:"H5Dget_space.vi"("obj (.)"=w829, "ref in"=w836) -> ("error out"=w843:errorcluster, "space out"=w838:T1)  [unwired: 8 in]
                      n187 = call <vilib>:"H5Sselect_simple.vi"("error in (no error)"=w843, "count"=w831, "start"=w830, "space in"=w838) -> ("error out"=w842:errorcluster, "space out"=w841:T1)  [unwired: 6 in]
                      n188 = xnode "H5Dwrite.xnode"("dataset name"=w829, "error in (no error)"=w842, "data"=w834, "file space"=w841, "ref in"=w836) -> ("error out"=w839:errorcluster)  [unwired: 2 in, 2 out]
                      n189 = call <vilib>:"H5Sclose.vi"("error in (no error)"=w839, "space in"=w838) -> ("error out"=w840:errorcluster)  [unwired: 9 in]
                      n190 = Unbundle By Name(w840) -> ("status"=w837:bool)
                      n191 = case shown="True" w837 {
                        tunnel: w836 -> [w845 _]
                        tunnel: [w845 w847] -> w835
                        tunnel: w833 -> [w844 w848]
                        tunnel: [w844 w846] -> w832
                        frame False {
                        }
                        frame True {
                          n192 = call "CloseOpenRef.vi"("Exp_params"=w848) -> ("Exp_params_out"=w846:T3, "group out"=w847:T1)  [unwired: 1 in]
                        }
                      }
                    }
                  }
                }
                frame #1 {
                  n193 = Delete From Array(array=w876, length=w872, index (row)=w873) -> (deleted portion=w874:dbl[][], array with subset deleted=w875:dbl[][])  [unwired: 1 in]
                  n194 = Index Array(array=w870, index=0) -> (element=w868:u64)
                  n195 = Index Array(array=w880, index=3) -> (element=w879:T1)
                  n196 = while {
                    tunnel: w882 -> [w901]
                    tunnel: w879 -> [w900]
                    tunnel: w878 -> [w899]
                    tunnel: [w898] -> w877
                    shift-right: [w883] -> _
                    shift-left: w875 -> [w894]
                    tunnel: w870 -> [w891]
                    shift-right: [w892] -> _
                    shift-left: w871 -> [w890]
                    tunnel: w868 -> [w887]
                    tunnel: w867 -> [w886]
                    stop <- w893 stop-if-true
                    n197 = Array Size(array=w894) -> (size(s)=w897:i32[])
                    n198 = Index Array(array=w897, index=0) -> (element=w888:i32)
                    n199 = Greater?(x=w888, y=w887) -> (0:w895:bool)
                    n200 = case shown="True" w895 {
                      tunnel: w890 -> [w906 w921]
                      tunnel: w887 -> [_ w917]
                      tunnel: w894 -> [w908 w920]
                      tunnel: [w908 w919] -> w889
                      tunnel: [TRUE FALSE] -> w893
                      tunnel: [dbl[][] [] w910] -> w883
                      tunnel: [w906 w915] -> w892
                      tunnel: w888 -> [w903 _]
                      tunnel: w887 -> [_ w913]
                      tunnel: w886 -> [w902 w914]
                      tunnel: [w904 w911] -> w885
                      frame False {
                        n201 = Replace Array Subset(array=w902, new element=w903, index=0) -> (w904:i32[])
                      }
                      frame True {
                        n202 = Delete From Array(array=w920, length=w917, index (row)=0) -> (deleted portion=w919:dbl[][], array with subset deleted=w910:dbl[][])  [unwired: 1 in]
                        n203 = Add(x=w917, y=w921) -> (x+y=w915:u64)
                        n204 = Replace Array Subset(array=w914, new element=w913, index=0) -> (w911:i32[])
                      }
                    }
                    n205 = call "Count2Indexes.vi"("sweep_dim"=w891, "Count"=w890) -> ("Indexes"=w884:u64[])
                    n206 = for {
                      tunnel: w901 -> [w928] mode=indexing
                      tunnel: w889 -> [w930]
                      tunnel: w900 -> [w927]
                      tunnel: w899 -> [w926]
                      tunnel: [w925] -> w898
                      tunnel: w884 -> [w923]
                      tunnel: w885 -> [w924]
                      i -> [w922]
                      n207 = Index Array(array=w930, index (col)=w922) -> (element=w929:dbl[])  [unwired: 1 in]
                      n208 = while {
                        shift-right: [w936] -> _
                        shift-left: w929 -> [w936]
                        shift-right: [w933] -> _
                        shift-left: w928 -> [w933]
                        shift-right: [w937] -> _
                        shift-left: w927 -> [w938]
                        shift-right: [w934] -> w925
                        shift-left: w926 -> [w935]
                        shift-right: [w932] -> _
                        shift-left: w924 -> [w932]
                        shift-right: [w931] -> _
                        shift-left: w923 -> [w931]
                        tunnel: w924 -> [_]
                        stop <- w939 continue-if-true
                        n209 = call <vilib>:"H5Dget_space.vi"("obj (.)"=w933, "ref in"=w938) -> ("error out"=w945:errorcluster, "space out"=w940:T1)  [unwired: 8 in]
                        n210 = call <vilib>:"H5Sselect_simple.vi"("error in (no error)"=w945, "count"=w932, "start"=w931, "space in"=w940) -> ("error out"=w944:errorcluster, "space out"=w943:T1)  [unwired: 6 in]
                        n211 = xnode "H5Dwrite.xnode"("dataset name"=w933, "error in (no error)"=w944, "data"=w936, "file space"=w943, "ref in"=w938) -> ("error out"=w941:errorcluster)  [unwired: 2 in, 2 out]
                        n212 = call <vilib>:"H5Sclose.vi"("error in (no error)"=w941, "space in"=w940) -> ("error out"=w942:errorcluster)  [unwired: 9 in]
                        n213 = Unbundle By Name(w942) -> ("status"=w939:bool)
                        n214 = case shown="True" w939 {
                          tunnel: w938 -> [w947 _]
                          tunnel: [w947 w949] -> w937
                          tunnel: w935 -> [w946 w950]
                          tunnel: [w946 w948] -> w934
                          frame False {
                          }
                          frame True {
                            n215 = call "CloseOpenRef.vi"("Exp_params"=w950) -> ("Exp_params_out"=w948:T3, "group out"=w949:T1)  [unwired: 1 in]
                          }
                        }
                      }
                    }
                  }
                }
                frame #2 {
                  n216 = Unbundle By Name(w972) -> ("File Ref list"=w976:T1[])
                  n217 = Index Array(array=w976, index=3) -> (element=w974:T1)
                  n218 = for {
                    tunnel: w977 -> [w984] mode=indexing
                    tunnel: w971 -> [w986]
                    tunnel: w974 -> [w983]
                    tunnel: w969 -> [w982]
                    tunnel: w970 -> [w981]
                    tunnel: w972 -> [w980]
                    tunnel: [w979] -> _
                    tunnel: [w979] -> w973
                    i -> [w978]
                    n219 = Index Array(array=w986, index (col)=w978) -> (element=w985:dbl[])  [unwired: 1 in]
                    n220 = while {
                      shift-right: [w992] -> _
                      shift-left: w985 -> [w992]
                      shift-right: [w987] -> _
                      shift-left: w984 -> [w987]
                      shift-right: [w993] -> _
                      shift-left: w983 -> [w994]
                      shift-right: [w990] -> w979
                      shift-left: w980 -> [w991]
                      shift-right: [w989] -> _
                      shift-left: w982 -> [w989]
                      shift-right: [w988] -> _
                      shift-left: w981 -> [w988]
                      stop <- w995 continue-if-true
                      n221 = call <vilib>:"H5Dget_space.vi"("obj (.)"=w987, "ref in"=w994) -> ("error out"=w1001:errorcluster, "space out"=w996:T1)  [unwired: 8 in]
                      n222 = call <vilib>:"H5Sselect_simple.vi"("error in (no error)"=w1001, "count"=w989, "start"=w988, "space in"=w996) -> ("error out"=w1000:errorcluster, "space out"=w999:T1)  [unwired: 6 in]
                      n223 = xnode "H5Dwrite.xnode"("dataset name"=w987, "error in (no error)"=w1000, "data"=w992, "file space"=w999, "ref in"=w994) -> ("error out"=w997:errorcluster)  [unwired: 2 in, 2 out]
                      n224 = call <vilib>:"H5Sclose.vi"("error in (no error)"=w997, "space in"=w996) -> ("error out"=w998:errorcluster)  [unwired: 9 in]
                      n225 = Unbundle By Name(w998) -> ("status"=w995:bool)
                      n226 = case shown="True" w995 {
                        tunnel: w994 -> [w1003 _]
                        tunnel: [w1003 w1005] -> w993
                        tunnel: w991 -> [w1002 w1006]
                        tunnel: [w1002 w1004] -> w990
                        frame False {
                        }
                        frame True {
                          n227 = call "CloseOpenRef.vi"("Exp_params"=w1006) -> ("Exp_params_out"=w1004:T3, "group out"=w1005:T1)  [unwired: 1 in]
                        }
                      }
                    }
                  }
                }
              }
            }
          }
        }
      }
    }
  }
  "count out" <- w2
  "Exp_params out" <- w1
